vi "Cleanup.vi"(8 "error in (no error)":errorcluster, 11 "InMemoryUserProvider in":refnum<class "InMemoryUserProvider.lvclass">) -> (0 "error out":errorcluster)   [LabVIEW 2020, in "HTTP Server.lvlib" / "InMemoryUserProvider.lvclass"]
uses:
  InMemoryUserProvider.lvclass
  InMemoryUserProvider.lvclass/InMemoryUserProvider.ctl
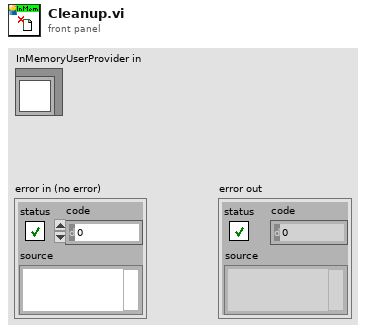
[diagram p1: front panel]
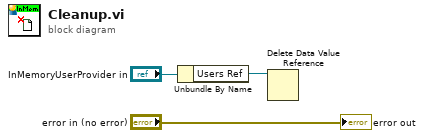
[diagram p0: block diagram]
diagram:
  n1 = Unbundle By Name("InMemoryUserProvider in") -> ("Users Ref"=w1:refnum<data-value>)
  n2 = Delete Data Value Reference(data value reference=w1) -> ()  [unwired: 1 in, 2 out]
  "error out" <- "error in (no error)"
